vi "fix default 2.vi"(10 "frekans index":dbl, 11 "default values":T1(array[cluster]) {"Kelvin Yk-1" format="%.4p"; "Wagner Yk-1" format="%.4p"; "1R Yk-1" format="%.4p"; "10R Yk-1" format="%.4p"; "Ana Denge Yk-1" format="%.4p"; "Kelvin Yk" format="%.4p"; "Wagner Yk" format="%.4p"; "1R Yk" format="%.4p"; "10R Yk" format="%.4p"; "Ana Denge Yk" format="%.4p"; "Kelvin Xk-1" format="%.4p"; "Wagner Xk-1" format="%.4p"; "1R Xk-1" format="%.4p"; "10R Xk-1" format="%.4p"; "Ana Denge Xk-1" format="%.4p"; "Kelvin Xk" format="%.4p"; "Wagner Xk" format="%.4p"; "1R Xk" format="%.4p"; "10R Xk" format="%.4p"; "Ana Denge Xk" format="%.4p"}) -> (3 "fix default":bool)   [LabVIEW 2014]
uses:
  DB_Global_4_kart-Test.vi
panel:
  in  "GPIB In":refnum<visa-resource-name>="GPIB0::8::INSTR"
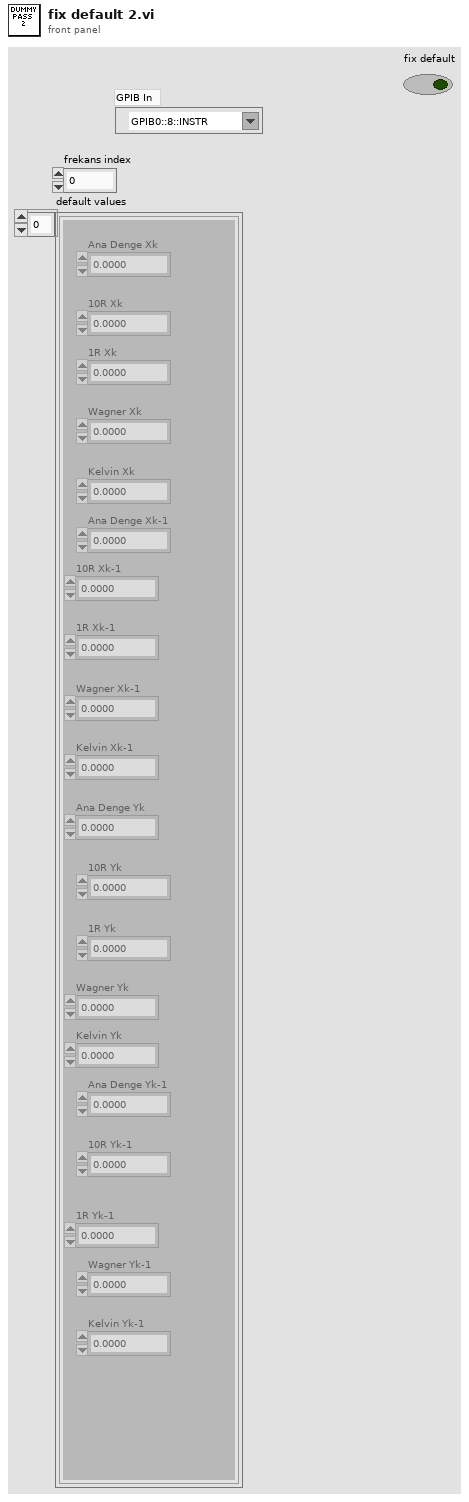
[diagram p1: front panel]
types:
  T1 = cluster{"Ana Denge Xk":dbl, "10R Xk ":dbl, "1R Xk ":dbl, "Wagner Xk":dbl, "Kelvin Xk ":dbl, "Ana Denge Xk-1":dbl, "10R Xk-1":dbl, "1R Xk-1":dbl, "Wagner Xk-1":dbl, "Kelvin Xk-1":dbl, "Ana Denge Yk":dbl, "10R Yk":dbl, "1R Yk":dbl, "Wagner Yk ":dbl, "Kelvin Yk ":dbl, "Ana Denge Yk-1":dbl, "10R Yk-1":dbl, "1R Yk-1":dbl, "Wagner Yk-1":dbl, "Kelvin Yk-1":dbl}[]
  T2 = cluster{"Ana Denge Xk":dbl, "10R Xk ":dbl, "1R Xk ":dbl, "Wagner Xk":dbl, "Kelvin Xk ":dbl, "Ana Denge Xk-1":dbl, "10R Xk-1":dbl, "1R Xk-1":dbl, "Wagner Xk-1":dbl, "Kelvin Xk-1":dbl, "Ana Denge Yk":dbl, "10R Yk":dbl, "1R Yk":dbl, "Wagner Yk ":dbl, "Kelvin Yk ":dbl, "Ana Denge Yk-1":dbl, "10R Yk-1":dbl, "1R Yk-1":dbl, "Wagner Yk-1":dbl, "Kelvin Yk-1":dbl}
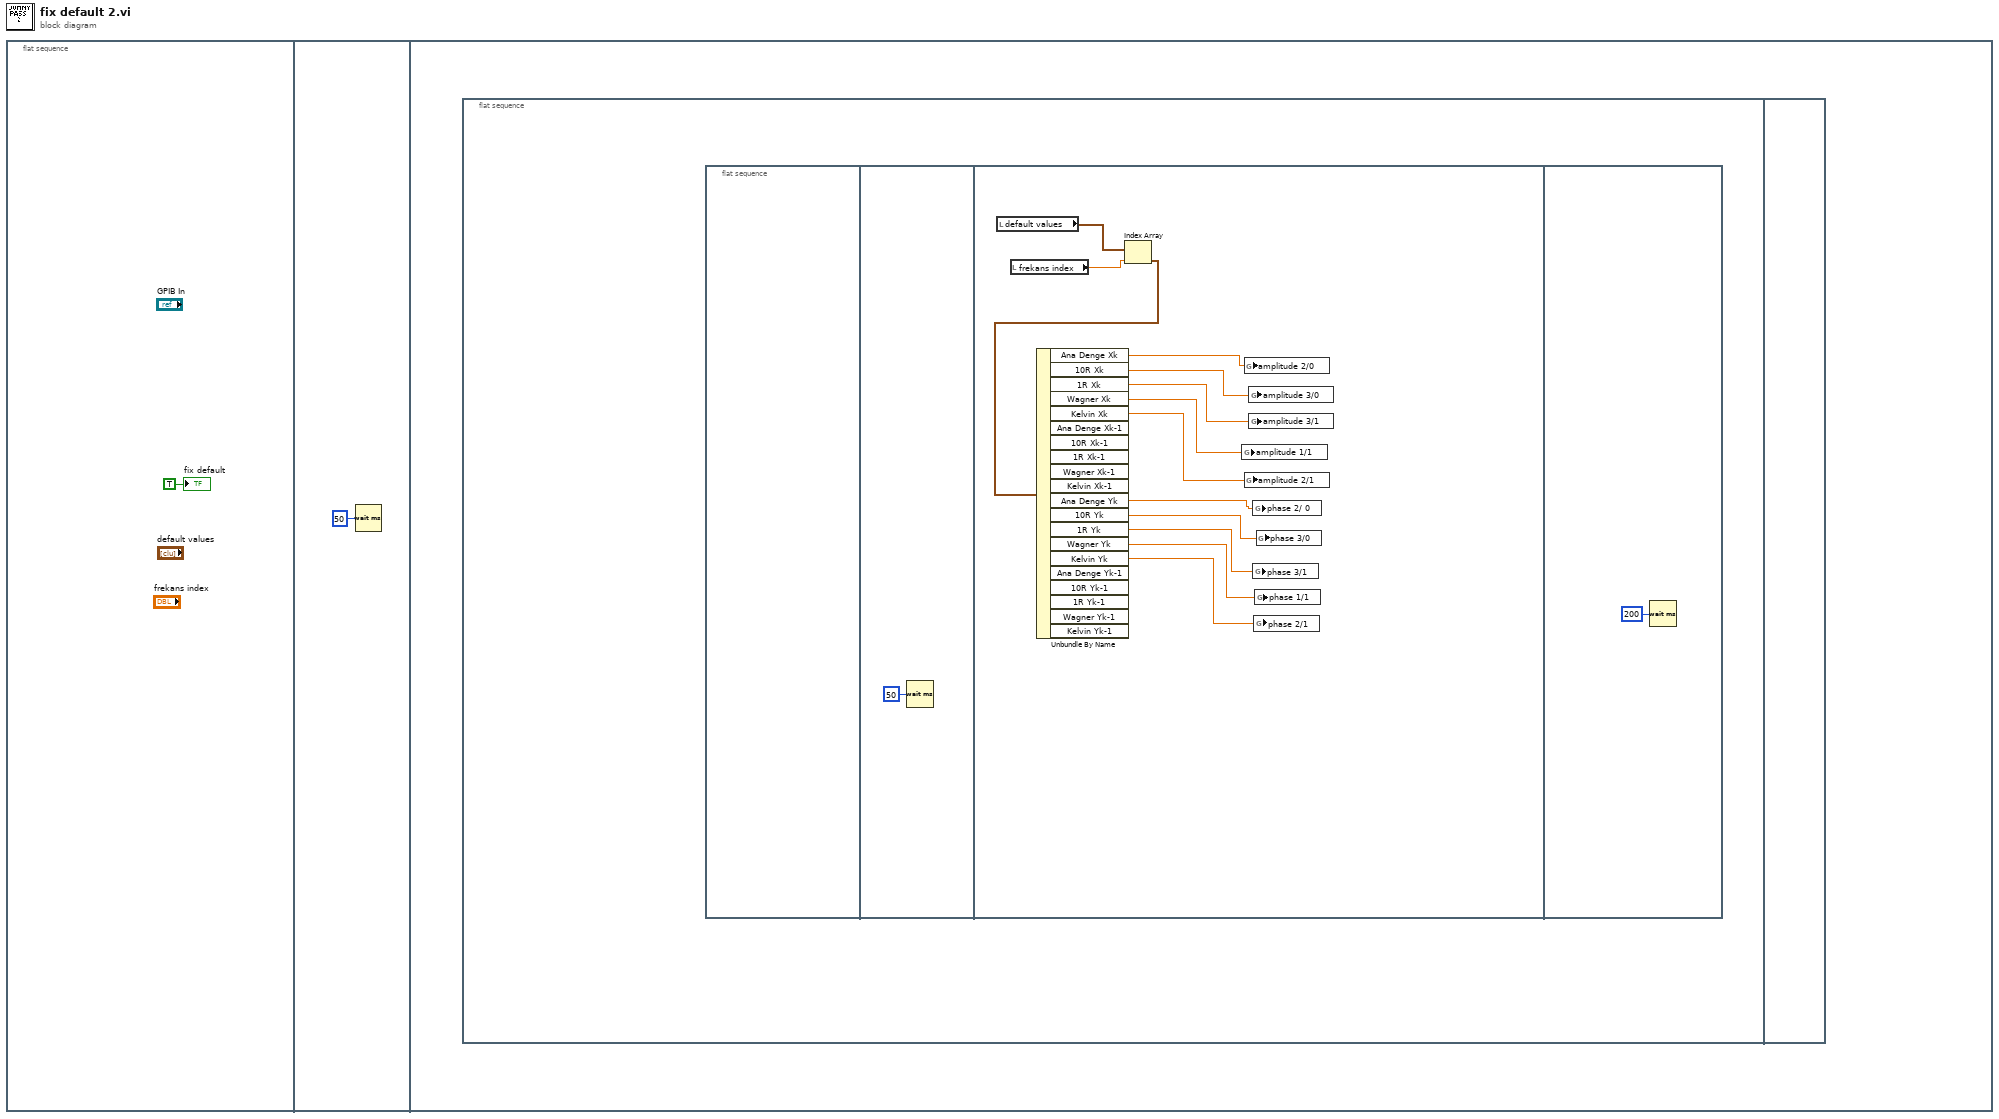
[diagram p0: block diagram]
diagram:
  n1 = flat-sequence {
    frame #0 {
      "fix default" <- TRUE ("fix default")
    }
    frame #1 {
      n2 = Wait (ms)(milliseconds to wait=u32 50) -> ()  [unwired: 1 out]
    }
    frame #2 {
      n3 = flat-sequence {
        frame #0 {
          n4 = flat-sequence {
            frame #0 {
            }
            frame #1 {
              n5 = Wait (ms)(milliseconds to wait=u32 50) -> ()  [unwired: 1 out]
            }
            frame #2 {
              n6 = local read "default values"() -> (w15:T1)
              n7 = local read "frekans index"() -> (w16:dbl)
              n8 = Index Array(array=w15, index=w16) -> (element=w14:T2)
              n9 = Unbundle By Name(w14) -> ("Ana Denge Xk"=w13:dbl, "10R Xk"=w12:dbl, "1R Xk"=w11:dbl, "Wagner Xk"=w10:dbl, "Kelvin Xk"=w9:dbl, "Ana Denge Yk"=w8:dbl, "10R Yk"=w7:dbl, "1R Yk"=w6:dbl, "Wagner Yk"=w5:dbl, "Kelvin Yk"=w4:dbl)  [unwired: 10 out]
              n10 = global write "DB_Global_4_kart-Test.vi" "amplitude 1/1"(w10) -> ()
              n11 = global write "DB_Global_4_kart-Test.vi" "amplitude 2/0"(w13) -> ()
              n12 = global write "DB_Global_4_kart-Test.vi" "amplitude 2/1"(w9) -> ()
              n13 = global write "DB_Global_4_kart-Test.vi" "amplitude 3/0"(w12) -> ()
              n14 = global write "DB_Global_4_kart-Test.vi" "amplitude 3/1"(w11) -> ()
              n15 = global write "DB_Global_4_kart-Test.vi" "phase 2/ 0"(w8) -> ()
              n16 = global write "DB_Global_4_kart-Test.vi" "phase 3/1"(w6) -> ()
              n17 = global write "DB_Global_4_kart-Test.vi" "phase 2/1"(w4) -> ()
              n18 = global write "DB_Global_4_kart-Test.vi" "phase 1/1"(w5) -> ()
              n19 = global write "DB_Global_4_kart-Test.vi" "phase 3/0"(w7) -> ()
            }
            frame #3 {
              n20 = Wait (ms)(milliseconds to wait=u32 200) -> ()  [unwired: 1 out]
            }
          }
        }
        frame #1 {
        }
      }
    }
  }
